vi "Create.vi"(8 "error in (no error)":errorcluster, 9 "Task ID":string, 10 "EnQr":refnum<class "Message Enqueuer.lvclass">) -> (0 "error out":errorcluster, 3 "DataLoggerAPI out":refnum<class "DataLoggerAPI.lvclass">)   [LabVIEW 2020, in "VolatusDataLogger.lvlib" / "DataLoggerAPI.lvclass"]
uses:
  DataLoggerAPI.lvclass
  <vilib>/ActorFramework/Message Enqueuer/Message Enqueuer.lvclass
  DataLoggerAPI.lvclass/DataLoggerAPI.ctl
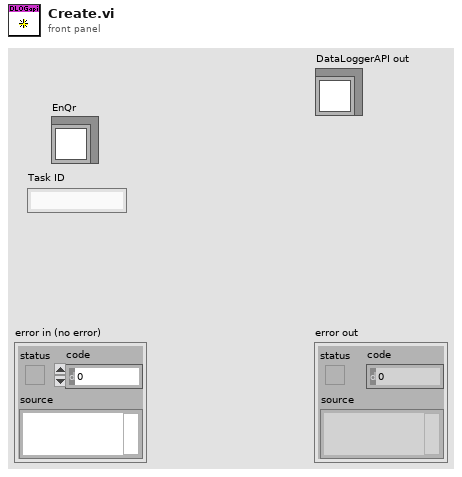
[diagram p1: front panel]
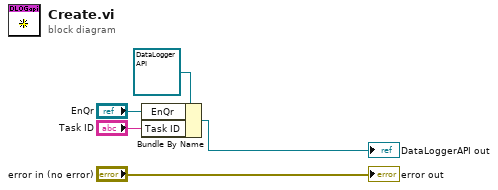
[diagram p0: block diagram]
diagram:
  n1 = Bundle By Name(cluster=refnum<class "DataLoggerAPI.lvclass"> refnum ("DataLoggerAPI in"), "EnQr"="EnQr", "Task ID"="Task ID") -> (→"DataLoggerAPI out":refnum<class "DataLoggerAPI.lvclass">)
  "error out" <- "error in (no error)"
